vi "Write Filename_ref.vi"(8 "error in":errorcluster, 10 "Filename_ref":refnum<vi>, 11 "Report Viewer in":refnum<class "Report Viewer.lvclass">) -> (0 "error out":errorcluster, 3 "Report Viewer out":refnum<class "Report Viewer.lvclass">)   [LabVIEW 2019, in "Report Viewer.lvlib" / "Report Viewer.lvclass"]
uses:
  Library/Report Viewer.lvclass
  Library/Report Viewer.lvclass/Report Viewer.ctl
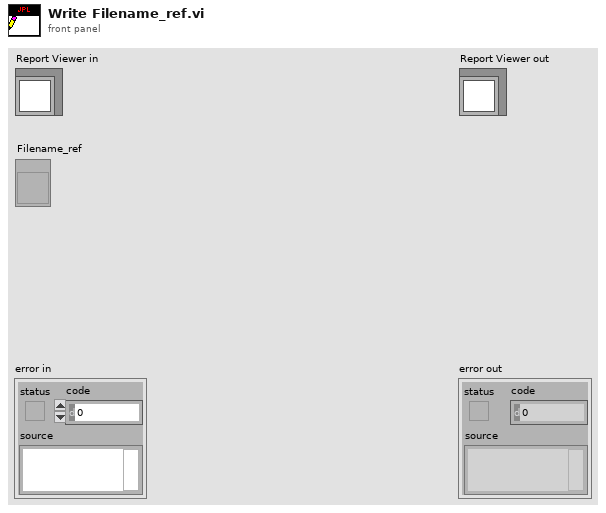
[diagram p1: front panel]
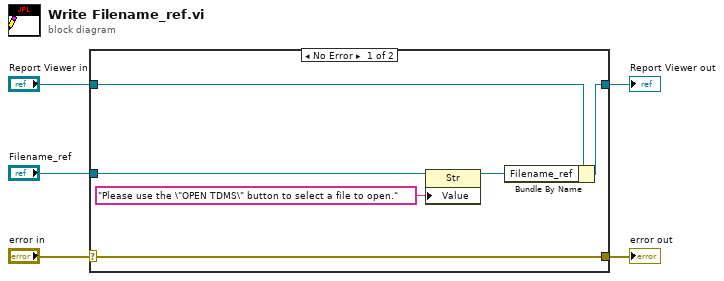
[diagram p0: block diagram]
diagram:
  n1 = case shown="No Error" "error in" {
    selector: "error in" -> [w11 w12]
    tunnel: [w11 w12] -> w4
    tunnel: [w9 w13] -> w2
    tunnel: "Report Viewer in" -> [w10 w13]
    tunnel: "Filename_ref" -> [w8 _]
    frame No Error {
      n2 = property class="Str"(reference=w8, "Value"="Please use the \"OPEN TDMS\" button to select a file to open.") -> (reference out=w7:refnum<vi>)  [unwired: 1 in, 1 out]
      n3 = Bundle By Name(cluster=w10, "Filename_ref"=w7) -> (w9:refnum<class "Report Viewer.lvclass">)
    }
    frame Error {
    }
  }
  "error out" <- w4
  "Report Viewer out" <- w2
